vi "Check exctraction cursors.vi"(8 "error in (no error)":errorcluster) -> (0 "error out":errorcluster, 1 "Cursors positions":T1, 3 "Extraction cursors at default positions":bool)   [LabVIEW 2013]
uses:
  Globals/gl_Time series viewer globals.vi
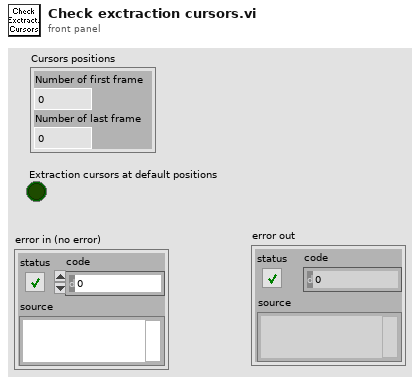
[diagram p1: front panel]
types:
  T1 = cluster{"Number of first frame":i32, "Number of last frame":i32}
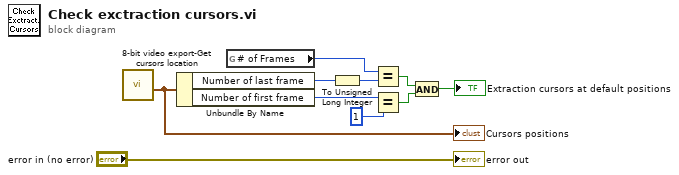
[diagram p0: block diagram]
diagram:
  n1 = call "8-bit video export-Get cursors location.vi"() -> ("Cursors location"=w10:T1)  [unwired: 11 in]
  "Cursors positions" <- w10
  n2 = Unbundle By Name(w10) -> ("Number of last frame"=w8:i32, "Number of first frame"=w7:i32)
  n3 = global read "gl_Time series viewer globals.vi" "# of Frames"() -> (w4:u32)
  n4 = To Unsigned Long Integer(number=w8) -> (unsigned 32bit integer=w9:u32)
  n5 = Equal?(x=w4, y=w9) -> (x = y?=w3:bool)
  n6 = Equal?(x=w7, y=1) -> (x = y?=w2:bool)
  n7 = And(x=w3, y=w2) -> (x .and. y?=→"Extraction cursors at default positions":bool)
  "error out" <- "error in (no error)"
